vi "FPGA_Scan_trigger_camera_synchro_laser_lines.vi"(3 "N Z positions":i32) -> ()   [LabVIEW 2015]
uses:
  <vilib>/rvi/Emulation/niFpgaGetClockAttributes.vi
  <vilib>/rvi/Emulation/niFpgaSctlEmulationGetInTimedLoop.vi
  <vilib>/rvi/Emulation/niFpgaEmulationReportErrorSimple.vi
  <vilib>/rvi/eio/common/nirviEmuTemplateMethod_errors.vi
  <vilib>/rvi/Emulation/niFpgaCriticalErrorInLSC.vi
  <vilib>/eio/EIONode/EIONode.xnode
panel:
  out "Images acquired":i32
  in  "Laser lines":i32[](array[numeric])=[0, 0, 0, 0, 0]
  in  "Laser power":sgl[](array[numeric])=[0.0, 0.0, 0.0, 0.0, 0.0]
  in  "N laser lines":i32
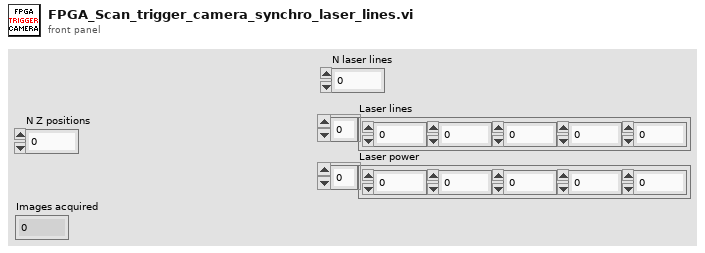
[diagram p1: front panel]
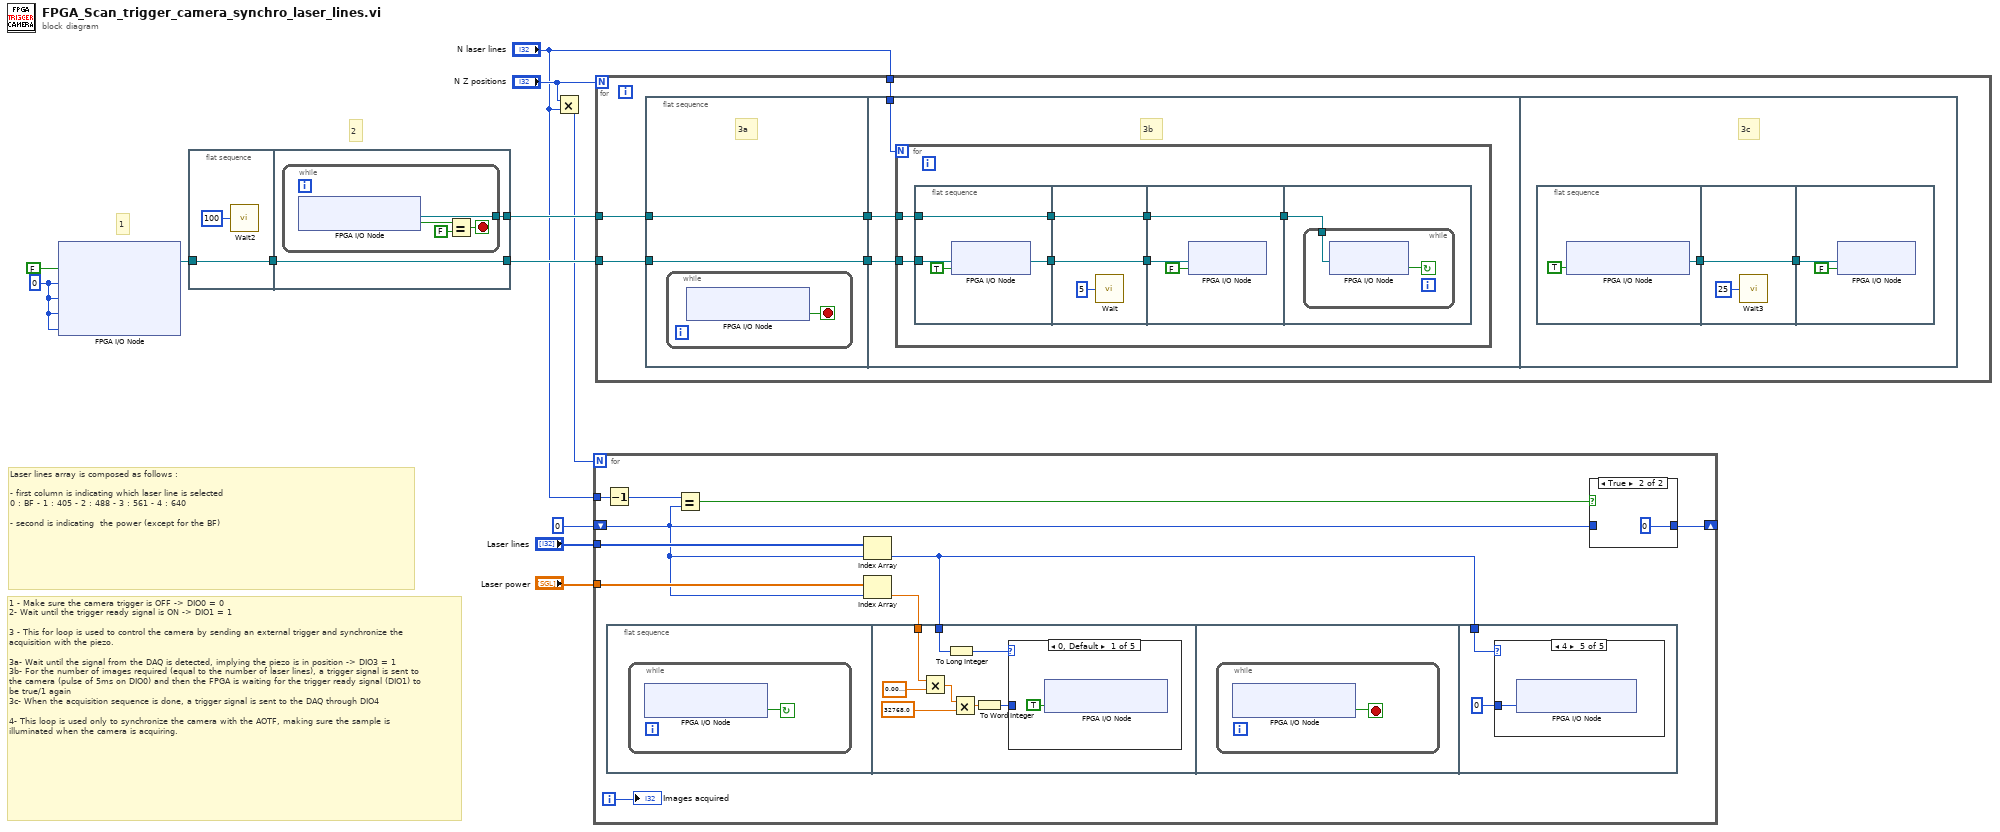
[diagram p0: block diagram]
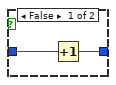
[diagram p2: hidden frame]
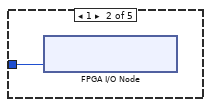
[diagram p3: hidden frame]
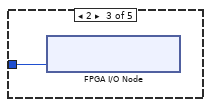
[diagram p4: hidden frame]
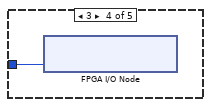
[diagram p5: hidden frame]
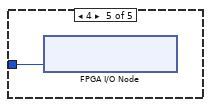
[diagram p6: hidden frame]
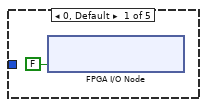
[diagram p7: hidden frame]
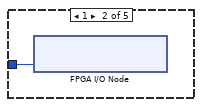
[diagram p8: hidden frame]
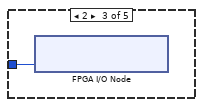
[diagram p9: hidden frame]
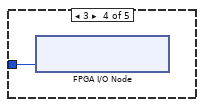
[diagram p10: hidden frame]
diagram:
  w1 = i16 0 ("Connector0/AO0")
  # "2"
  # "1"
  # "1 - Make sure the camera trigger is OFF -> DIO0 = 0\n2- Wait until the trigger ready signal is ON -> DIO1 = 1\n\n3 - This for loop is used to control the camera by sending an external trigger and synchronize the acquisition with the piezo.\n\n3a- Wait until the signal from the DAQ is detected, implying the piezo is in position -> DIO3 = 1 \n3b- For the number of images required (equal to the number of laser lines), a trigger signal is sent to the camera (pulse of 5ms on DIO0) and then the FPGA is waiting for the trigger ready signal (DIO1) to be true/1 again\n3c- When the acquisition sequence is done, a trigger signal is sent to the DAQ through DIO4\n\n4- This loop is used only to synchronize the camera with the AOTF, making sure the sample is illuminated when the camera is acquiring."
  # "Laser lines array is composed as follows :\n\n- first column is indicating which laser line is selected \n0 : BF - 1 : 405 - 2 : 488 - 3 : 561 - 4 : 640\n\n- second is indicating  the power (except for the BF)"
  n1 = xnode "FPGA I/O Node"("Connector0/DIO0"=FALSE, "Connector0/AO0"=w1, "Connector0/AO1"=w1, "Connector0/AO2"=w1, "Connector0/AO3"=w1) -> ("FPGA I/O Out"=w11:refnum<k21>)  [unwired: 5 in, 4 out]
  n2 = flat-sequence {
    tunnel: w11 -> [w14]
    tunnel: [w14] -> w10
    tunnel: w10 -> [w16]
    tunnel: [w16] -> w9
    tunnel: [w15] -> w8
    frame #0 {
      n3 = call "Wait2"("Count(uSec)"=u32 100 ("Count(mSec)")) -> ()  [unwired: 1 out]
    }
    frame #1 {
      n4 = while {
        tunnel: [w20] -> w15
        stop <- w17 stop-if-true
        n5 = xnode "FPGA I/O Node"() -> ("Connector0/DIO1"=w19:bool, "FPGA I/O Out"=w20:refnum<k21>)  [unwired: 1 in]
        n6 = Equal?(x=w19, y=FALSE) -> (x = y?=w17:bool)
      }
    }
  }
  n7 = Multiply(x="N Z positions", y="N laser lines") -> (x*y=w3:i32)
  n8 = for {
    N: w3 -> [_]
    shift-right: [w28] -> _
    shift-left: 0 -> [w25]
    tunnel: "Laser lines" -> [w27]
    tunnel: "Laser power" -> [w26]
    tunnel: "N laser lines" -> [w23]
    i -> [w21]
    n9 = Decrement(x=w23) -> (x-1=w22:i32)
    n10 = flat-sequence {
      tunnel: w30 -> [w37]
      tunnel: w24 -> [w36]
      tunnel: w30 -> [w49]
      frame #0 {
        n11 = while {
          stop <- w34 continue-if-true
          n12 = xnode "FPGA I/O Node"() -> ("Connector0/DIO2"=w34:bool)  [unwired: 1 in, 1 out]
        }
      }
      frame #1 {
        n13 = Multiply(x=w36, y=sgl 0.01) -> (x*y=w35:sgl)
        n14 = To Long Integer(number=w37) -> (32bit integer=w42:i32)
        n15 = Multiply(x=w35, y=sgl 32768.0) -> (x*y=w39:sgl)
        n16 = To Word Integer(number=w39) -> (16bit integer=w38:i16)
        n17 = case shown="0, Default" w42 {
          tunnel: w38 -> [_ w44 w45 w46 w47]
          frame 0, Default {
            n18 = xnode "FPGA I/O Node"("Connector0/DIO5"=TRUE) -> ()  [unwired: 1 in, 1 out]
          }
          frame 1 {
            n19 = xnode "FPGA I/O Node"("Connector0/AO2"=w44) -> ()  [unwired: 1 in, 1 out]
          }
          frame 2 {
            n20 = xnode "FPGA I/O Node"("Connector0/AO3"=w45) -> ()  [unwired: 1 in, 1 out]
          }
          frame 3 {
            n21 = xnode "FPGA I/O Node"("Connector0/AO0"=w46) -> ()  [unwired: 1 in, 1 out]
          }
          frame 4 {
            n22 = xnode "FPGA I/O Node"("Connector0/AO1"=w47) -> ()  [unwired: 1 in, 1 out]
          }
        }
      }
      frame #2 {
        n23 = while {
          stop <- w48 stop-if-true
          n24 = xnode "FPGA I/O Node"() -> ("Connector0/DIO2"=w48:bool)  [unwired: 1 in, 1 out]
        }
      }
      frame #3 {
        n25 = case shown="4" w49 {
          tunnel: i16 0 -> [_ w52 w53 w54 w55]
          frame 0, Default {
            n26 = xnode "FPGA I/O Node"("Connector0/DIO5"=FALSE) -> ()  [unwired: 1 in, 1 out]
          }
          frame 1 {
            n27 = xnode "FPGA I/O Node"("Connector0/AO2"=w52) -> ()  [unwired: 1 in, 1 out]
          }
          frame 2 {
            n28 = xnode "FPGA I/O Node"("Connector0/AO3"=w53) -> ()  [unwired: 1 in, 1 out]
          }
          frame 3 {
            n29 = xnode "FPGA I/O Node"("Connector0/AO0"=w54) -> ()  [unwired: 1 in, 1 out]
          }
          frame 4 {
            n30 = xnode "FPGA I/O Node"("Connector0/AO1"=w55) -> ()  [unwired: 1 in, 1 out]
          }
        }
      }
    }
    n31 = Equal?(x=w22, y=w25) -> (x = y?=w29:bool)
    n32 = Index Array(array=w27, index=w25) -> (element=w30:i32)
    n33 = Index Array(array=w26, index=w25) -> (element=w24:sgl)
    n34 = case shown="True" w29 {
      tunnel: w25 -> [w32 _]
      tunnel: [w31 0] -> w28
      frame False {
        n35 = Increment(x=w32) -> (x+1=w31:i32)
      }
      frame True {
      }
    }
    "Images acquired" <- w21
  }
  n36 = for {
    N: "N Z positions" -> [_]
    tunnel: w9 -> [w59]
    tunnel: w8 -> [w60]
    tunnel: "N laser lines" -> [w56]
    n37 = flat-sequence {
      tunnel: w59 -> [w61]
      tunnel: w60 -> [w62]
      tunnel: [w62] -> w58
      tunnel: [w61] -> w57
      tunnel: w58 -> [w66]
      tunnel: w57 -> [w65]
      tunnel: w56 -> [w64]
      frame #0 {
        # "3a"
        n38 = while {
          stop <- w63 stop-if-true
          n39 = xnode "FPGA I/O Node"() -> ("Connector0/DIO3"=w63:bool)  [unwired: 1 in, 1 out]
        }
      }
      frame #1 {
        # "3b"
        n40 = for {
          N: w64 -> [_]
          tunnel: w66 -> [w68]
          tunnel: w65 -> [w67]
          n41 = flat-sequence {
            tunnel: [w76] -> w73
            tunnel: [w74] -> w72
            tunnel: w67 -> [w75]
            tunnel: w68 -> [w74]
            tunnel: w73 -> [w79]
            tunnel: [w79] -> w71
            tunnel: [w78] -> w70
            tunnel: w72 -> [w78]
            tunnel: w71 -> [w82]
            tunnel: [w81] -> w69
            tunnel: w70 -> [w81]
            tunnel: w69 -> [w84]
            frame #0 {
              n42 = xnode "FPGA I/O Node"("I/O Item"=TRUE ("Connector0/DIO0"), "FPGA I/O In"=w75) -> ("FPGA I/O Out"=w76:refnum<k21>)
            }
            frame #1 {
              n43 = call "Wait"("Count(mSec)"=u32 5) -> ()  [unwired: 1 out]
            }
            frame #2 {
              n44 = xnode "FPGA I/O Node"("I/O Item"=FALSE ("Connector0/DIO0"), "FPGA I/O In"=w82) -> ()  [unwired: 1 out]
            }
            frame #3 {
              n45 = while {
                tunnel: w84 -> [w86]
                stop <- w85 continue-if-true
                n46 = xnode "FPGA I/O Node"("FPGA I/O In"=w86) -> ("I/O Item"=w85:bool)  [unwired: 1 out]
              }
            }
          }
        }
      }
      frame #2 {
        # "3c"
        n47 = flat-sequence {
          tunnel: [w90] -> w88
          tunnel: w88 -> [w91]
          tunnel: [w91] -> w87
          tunnel: w87 -> [w93]
          frame #0 {
            n48 = xnode "FPGA I/O Node"("Connector0/DIO4"=TRUE) -> ("FPGA I/O Out"=w90:refnum<k21>)  [unwired: 1 in]
          }
          frame #1 {
            n49 = call "Wait3"("Count(mSec)"=u32 25) -> ()  [unwired: 1 out]
          }
          frame #2 {
            n50 = xnode "FPGA I/O Node"("I/O Item"=FALSE ("Connector0/DIO0"), "FPGA I/O In"=w93) -> ()  [unwired: 1 out]
          }
        }
      }
    }
  }
